vi "A0C23-Word to number.vi"(11 "Word":string) -> (3 "Number":string)   [LabVIEW 2021]
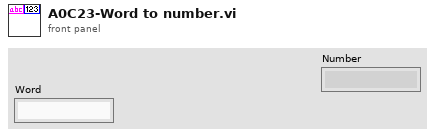
[diagram p1: front panel]
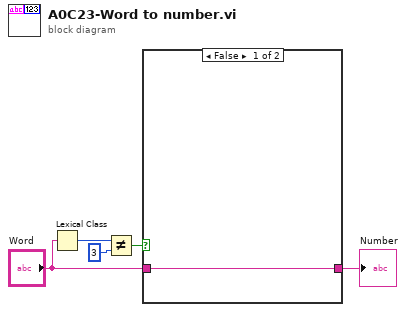
[diagram p0: block diagram]
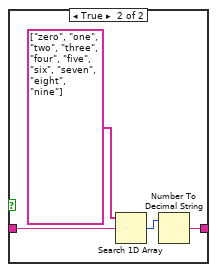
[diagram p2: hidden frame]
diagram:
  n1 = Lexical Class(1:"Word") -> (0:w2:i16)
  n2 = Not Equal?(x=w2, y=i16 3) -> (x != y?=w4:bool)
  n3 = case shown="False" w4 {
    tunnel: "Word" -> [w6 w9]
    tunnel: [w6 w8] -> w1
    frame False {
    }
    frame True {
      n4 = Search 1D Array(1D array=string[] ["zero", "one", "two", "three", "four", "five", "six", "seven", "eight", "nine"], element=w9) -> (index of element=w7:i32)  [unwired: 1 in]
      n5 = Number To Decimal String(number=w7) -> (decimal integer string=w8:string)  [unwired: 1 in]
    }
  }
  "Number" <- w1
